vi "VI_principal.vi"() -> ()   [LabVIEW 2024]
uses:
  <vilib>/LabVIEW Open Source Project/Epoch Date & Time/epoch.UNIX/Epoch.UNIX.lvclass
panel:
  in  "Tab Control":enum32{"Page 1", "Page 2", "Page 3"}(tab)
  out "Waveform Chart 3":waveform(dbl)(graph)
  out "output waveform":waveform(dbl)
  out "Waveform Chart 5":waveform(dbl)(graph)
  out "output waveform 2":waveform(dbl)
  out "Waveform Chart 7":waveform(dbl)(graph)
  out "output waveform 3":waveform(dbl)
  out "Waveform Chart 6":waveform(dbl)(graph)
  out "Waveform Chart 4":waveform(dbl)(graph)
  in  "stop":bool
  out "Waveform Chart 2":waveform(dbl)(graph)
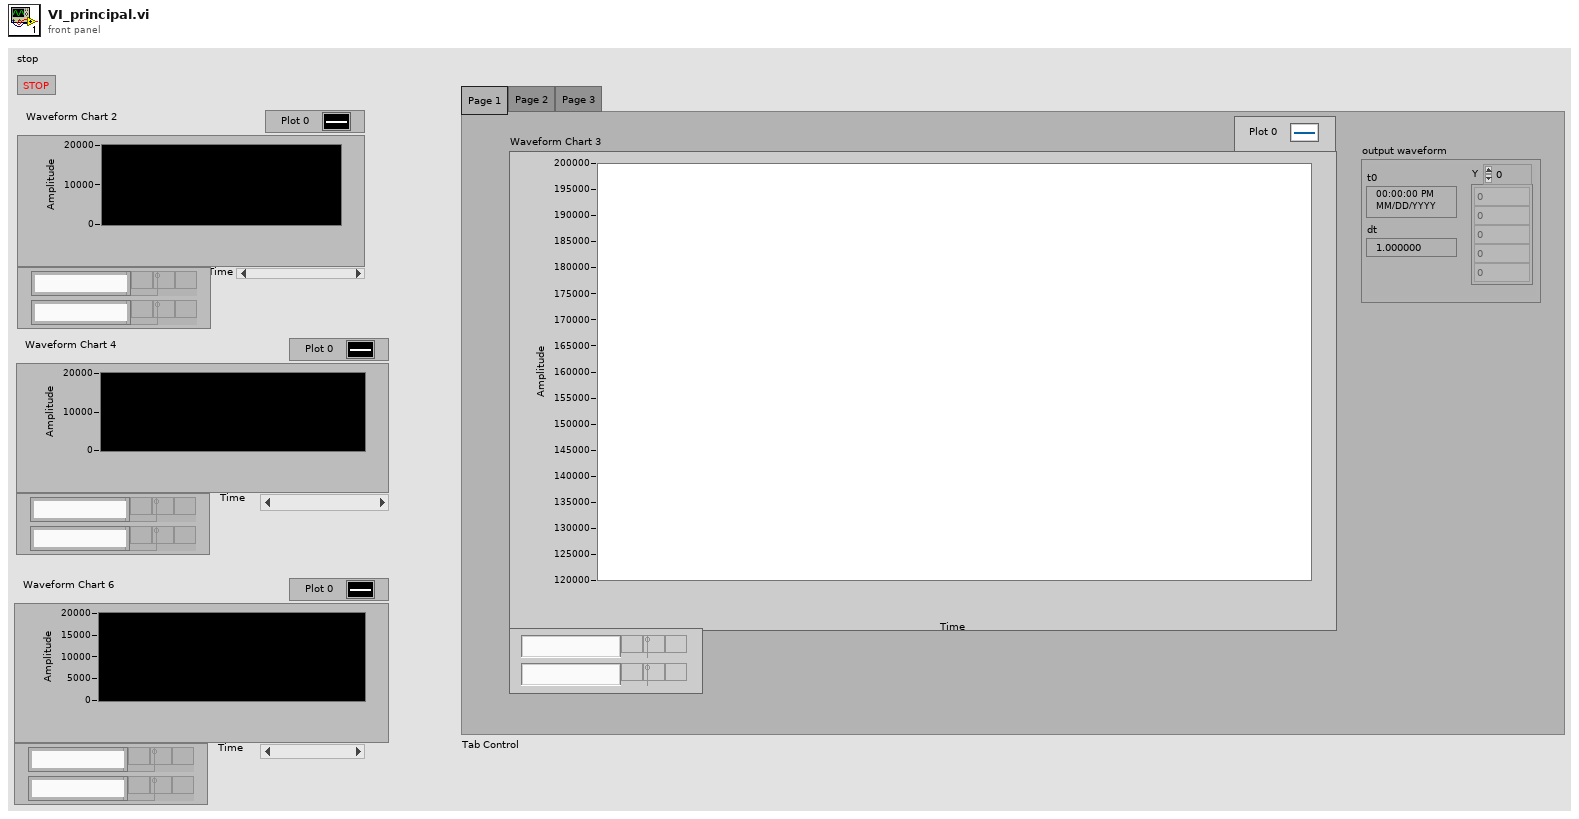
[diagram p1: front panel]
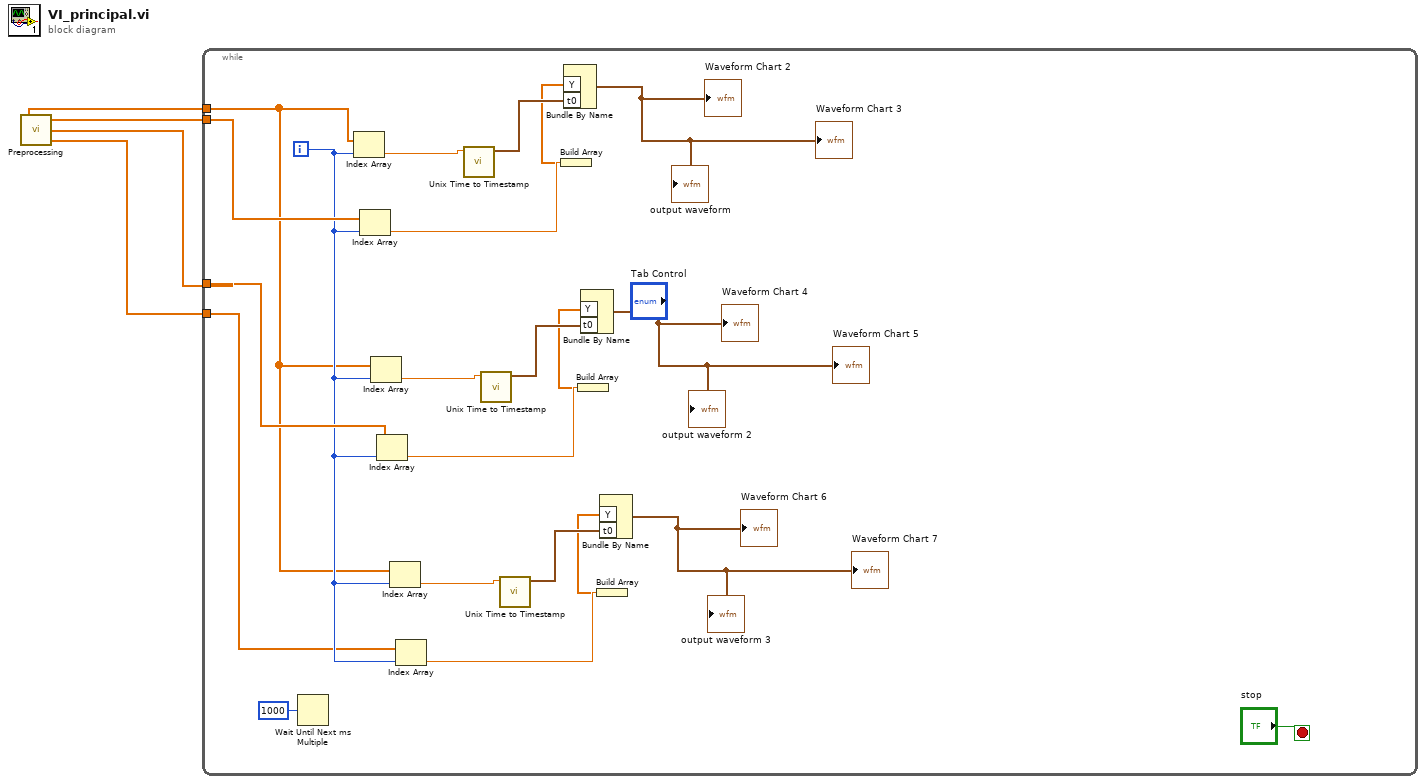
[diagram p0: block diagram]
diagram:
  n1 = call "Preprocessing.vi"() -> ("Timestamp"=w3:dbl[], "Potência instantänea A"=w4:dbl[], "Potência Ativa B"=w2:dbl[], "Potência Ativa C"=w1:dbl[])
  n2 = while {
    tunnel: w4 -> [w26]
    tunnel: w3 -> [w6]
    tunnel: w2 -> [w13]
    tunnel: w1 -> [w5]
    i -> [w7]
    stop <- "stop" stop-if-true
    n3 = Wait Until Next ms Multiple(millisecond multiple=u32 1000) -> ()  [unwired: 1 out]
    n4 = Index Array(array=w6, index=w7) -> (element=w25:dbl)
    n5 = Index Array(array=w26, index=w7) -> (element=w23:dbl)
    n6 = Index Array(array=w6, index=w7) -> (element=w18:dbl)
    n7 = Index Array(array=w13, index=w7) -> (element=w16:dbl)
    n8 = Index Array(array=w6, index=w7) -> (element=w12:dbl)
    n9 = Index Array(array=w5, index=w7) -> (element=w10:dbl)
    n10 = call <vilib>:"Unix Time to Timestamp.vi"("Unix Time (s)"=w25) -> ("Timestamp"=w24:timestamp)  [unwired: 9 in, 1 out]
    n11 = call <vilib>:"Unix Time to Timestamp.vi"("Unix Time (s)"=w18) -> ("Timestamp"=w17:timestamp)  [unwired: 9 in, 1 out]
    n12 = call <vilib>:"Unix Time to Timestamp.vi"("Unix Time (s)"=w12) -> ("Timestamp"=w11:timestamp)  [unwired: 9 in, 1 out]
    n13 = Build Array(w23) -> (w22:dbl[])
    n14 = Bundle By Name("Y"=w22, "t0"=w24) -> (→"output waveform" →"Waveform Chart 2" →"Waveform Chart 3":waveform(dbl))  [unwired: 1 in]
    n15 = Build Array(w16) -> (w15:dbl[])
    n16 = Bundle By Name("Y"=w15, "t0"=w17) -> (→"output waveform 2" →"Waveform Chart 4" →"Waveform Chart 5":waveform(dbl))  [unwired: 1 in]
    n17 = Build Array(w10) -> (w9:dbl[])
    n18 = Bundle By Name("Y"=w9, "t0"=w11) -> (→"output waveform 3" →"Waveform Chart 6" →"Waveform Chart 7":waveform(dbl))  [unwired: 1 in]
  }
